vi "Function.vi"(8 "error in (no error)":errorcluster, 10 "Value":dbl, 11 "Two Terminal in":refnum<class "Invert_CPLX_SGL.lvclass">) -> (0 "error out":errorcluster, 2 "Result":dbl, 3 "Two Terminal out":refnum<class "Invert_CPLX_SGL.lvclass">)   [LabVIEW 2021, in "Invert_CPLX_SGL.lvclass"]
uses:
  Invert_CPLX_SGL.lvclass
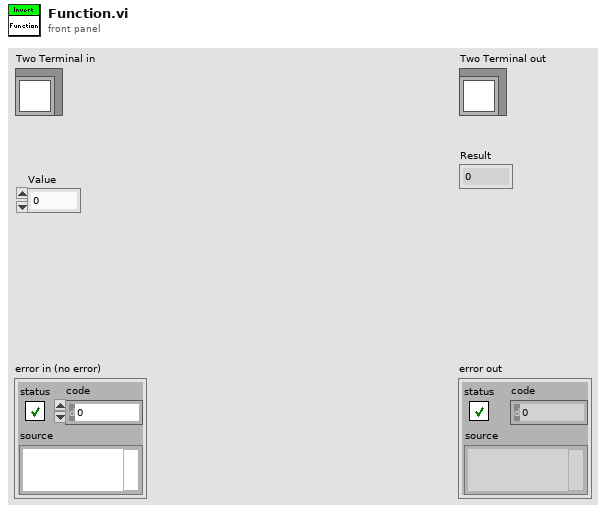
[diagram p1: front panel]
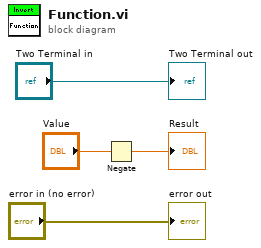
[diagram p0: block diagram]
diagram:
  n1 = Negate(x="Value") -> (-x=→"Result":dbl)
  "error out" <- "error in (no error)"
  "Two Terminal out" <- "Two Terminal in"
